vi "Pressure Alarm v1.vi"() -> ()   [LabVIEW 2013]
uses:
  <vilib>/measure/madcrms.llb/Basic Averaged DC-RMS for 1 Chan.vi
  <vilib>/express/express shared/transition.llb/Dynamic To Waveform Array.vi
  <vilib>/express/express signal manip/GetorSetDDTAttributes/Set DDT Attributes/SetT0.vi
  <vilib>/express/express shared/transition.llb/Waveform Array To Dynamic.vi
  <vilib>/express/express signal manip/GetorSetDDTAttributes/Set DDT Attributes/Set DDT Properties.xnode
  <vilib>/measure/NI_MAPro.lvlib
panel:
  out "Stalled 2":bool
  out "Waveform Chart 2":dbl(graph)
  out "Waveform Chart":dbl(graph)
  out "Stalled":bool
  in  "?":bool
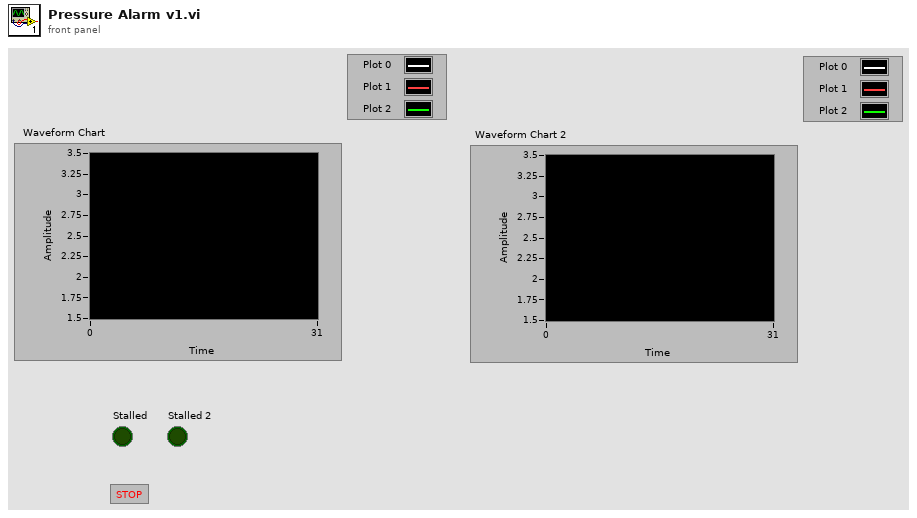
[diagram p1: front panel]
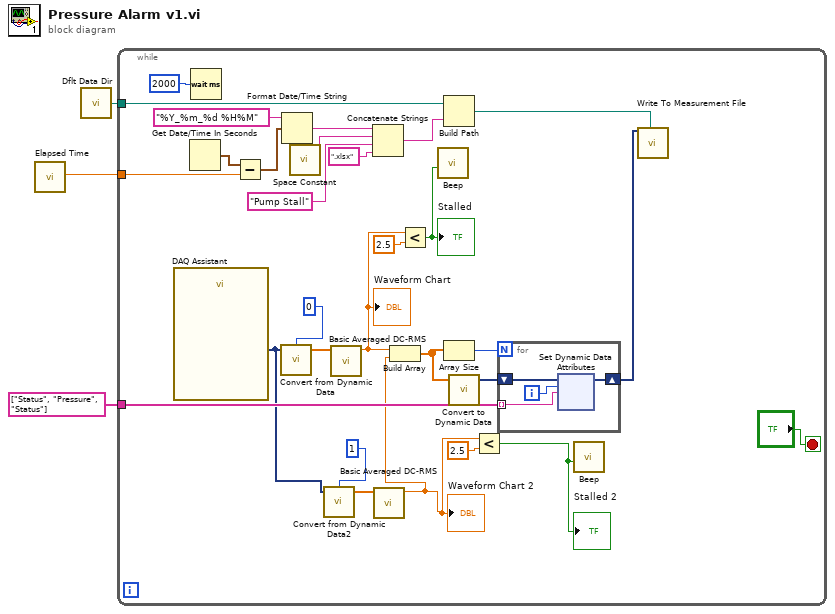
[diagram p0: block diagram]
diagram:
  n1 = call "Elapsed Time"() -> ("Elapsed Time (s)"=w3:dbl)  [unwired: 12 in, 7 out]
  n2 = call <vilib>:"Dflt Data Dir.vi"() -> ("App:Default Data Directory"=w2:path)
  n3 = while {
    tunnel: w3 -> [w28]
    tunnel: w2 -> [w19]
    tunnel: string[] ["Status", "Pressure", "Status"] ("Array") -> [w16]
    stop <- "?" stop-if-true
    n4 = call "DAQ Assistant"() -> ("data"=w7:dynamicdata)  [unwired: 17 in, 2 out]
    n5 = Get Date/Time In Seconds() -> (seconds since 1Jan1904=w29:timestamp)
    n6 = Wait (ms)(milliseconds to wait=2000) -> ()  [unwired: 1 out]
    n7 = Subtract(x=w29, y=w28) -> (x-y=w26:timestamp)
    n8 = call "Convert from Dynamic Data"("Dynamic Data Type"=w7, "Channel"=0) -> ("Array"=w11:dbl[])  [unwired: 2 in]
    n9 = Format Date/Time String(time format string (%c)="%Y_%m_%d %H%M", seconds (now)=w26) -> (date/time string=w24:string)  [unwired: 1 in]
    n10 = call <vilib>:"Space Constant.vi"() -> ("String"=w23:string)
    n11 = call "Convert from Dynamic Data2"("Dynamic Data Type"=w7, "Channel"=1) -> ("Array"=w9:dbl[])  [unwired: 2 in]
    n12 = call-poly <vilib>:"Basic Averaged DC-RMS.vi"("signal in"=w11) -> ("DC value"=w12:dbl)  [unwired: 7 in, 3 out]
    "Waveform Chart" <- w12
    n13 = Concatenate Strings(w24, w23, "Pump Stall" ("string"), ".xlsx" ("string")) -> (w21:string)
    n14 = call-poly <vilib>:"Basic Averaged DC-RMS.vi"("signal in"=w9) -> ("DC value"=w4:dbl)  [unwired: 7 in, 3 out]
    "Waveform Chart 2" <- w4
    n15 = Build Array(w12, w4) -> (w18:dbl[])
    n16 = Less?(x=w12, y=2.5) -> (x < y?=w13:bool)
    "Stalled" <- w13
    n17 = call <vilib>:"Beep.vi"("use system alert? (T)"=w13) -> ()  [unwired: 11 in]
    n18 = Build Path(base path=w19, name or relative path=w21) -> (appended path=w25:path)
    n19 = Array Size(array=w18) -> (size(s)=w17:i32)
    n20 = call "Convert to Dynamic Data"("Array"=w18) -> ("Dynamic Data Type"=w14:dynamicdata)  [unwired: 3 in]
    n21 = Less?(x=w4, y=2.5) -> (x < y?=w5:bool)
    "Stalled 2" <- w5
    n22 = for {
      N: w17 -> [_]
      tunnel: w16 -> [w35] mode=indexing
      shift-right: [w34] -> w15
      shift-left: w14 -> [w33]
      i -> [w36]
      n23 = xnode ("Set Dynamic Data Attributes")("Signals In"=w33, "Signal Index"=w36, "Signal Name"=w35) -> ("Signals Out"=w34:dynamicdata)  [unwired: 1 in, 1 out]
    }
    n24 = call <vilib>:"Beep.vi"("use system alert? (T)"=w5) -> ()  [unwired: 11 in]
    n25 = call "Write To Measurement File"("Signals"=w15, "Filename"=w25) -> ()  [unwired: 15 in, 3 out]
  }
